vi "Kaelus PFE Release.vi"(7 "Kaelus PFE":T1, 8 "error in (no error)":errorcluster, 11 "DAQmx Dev Name (FEModule)":string) -> (0 "error out":errorcluster {"code" format="%.0x"})   [LabVIEW 2011]
uses:
  TypeDefs/Kaelus PFE Instrument Info.ctl
  BPIMCore EXT/WebEngine/LIB/HW Global D.vi
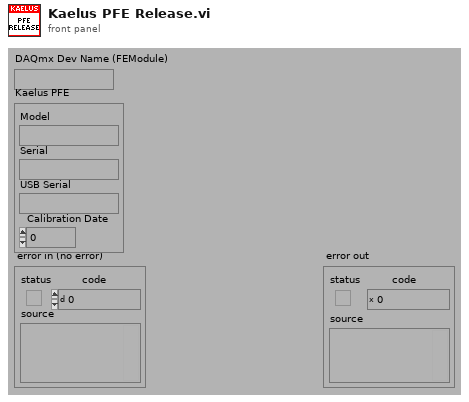
[diagram p1: front panel]
types:
  T1 = typedef "Kaelus PFE Instrument Info.ctl" = cluster{"Model":string, "Serial":string, "USB Serial":string, "Calibration Date":dbl}
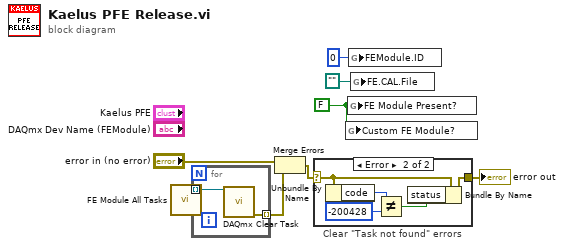
[diagram p0: block diagram]
diagram:
  w6 = FALSE ("FE Module Present?")
  n1 = call "FE Module All Tasks.vi"() -> ("Task Names"=w7:refnum<k21>[])  [unwired: 4 out]
  n2 = for {
    tunnel: [w10] -> w3 mode=indexing
    tunnel: w7 -> [w9] mode=indexing
    n3 = call <vilib>:"DAQmx Clear Task.vi"("task in"=w9) -> ("error out"=w10:errorcluster)  [unwired: 1 in, 13 out]
  }
  n4 = Merge Errors("error in (no error)", w3) -> (w2:errorcluster)
  n5 = case "Clear \"Task not found\" errors" shown="Error" w2 {
    selector: w2 -> [w11 w14]
    tunnel: [w11 w12] -> w1
    frame No Error {
    }
    frame Error {
      n6 = Unbundle By Name(w14) -> ("code"=w16:i32)
      n7 = Not Equal?(x=w16, y=-200428) -> (x != y?=w13:bool)
      n8 = Bundle By Name(cluster=w14, "status"=w13) -> (w12:errorcluster)
    }
  }
  "error out" <- w1
  n9 = global write "HW Global D.vi" "Custom FE Module?"(w6) -> ()
  n10 = global write "HW Global D.vi" "FE Module Present?"(w6) -> ()
  n11 = global write "HW Global D.vi" "FEModule.ID"(u16 0 ("FEModule.ID")) -> ()
  n12 = global write "HW Global D.vi" "FE.CAL.File"(path "") -> ()
